vi "задача 3.1.vi"() -> ()   [LabVIEW 2019]
uses:
  <vilib>/Utility/file.llb/Read Delimited Spreadsheet (I64).vi
panel:
  out "Min":dbl
  out "Max":dbl
  in  "Path":path
  out "Waveform Chart":i64[](graph)
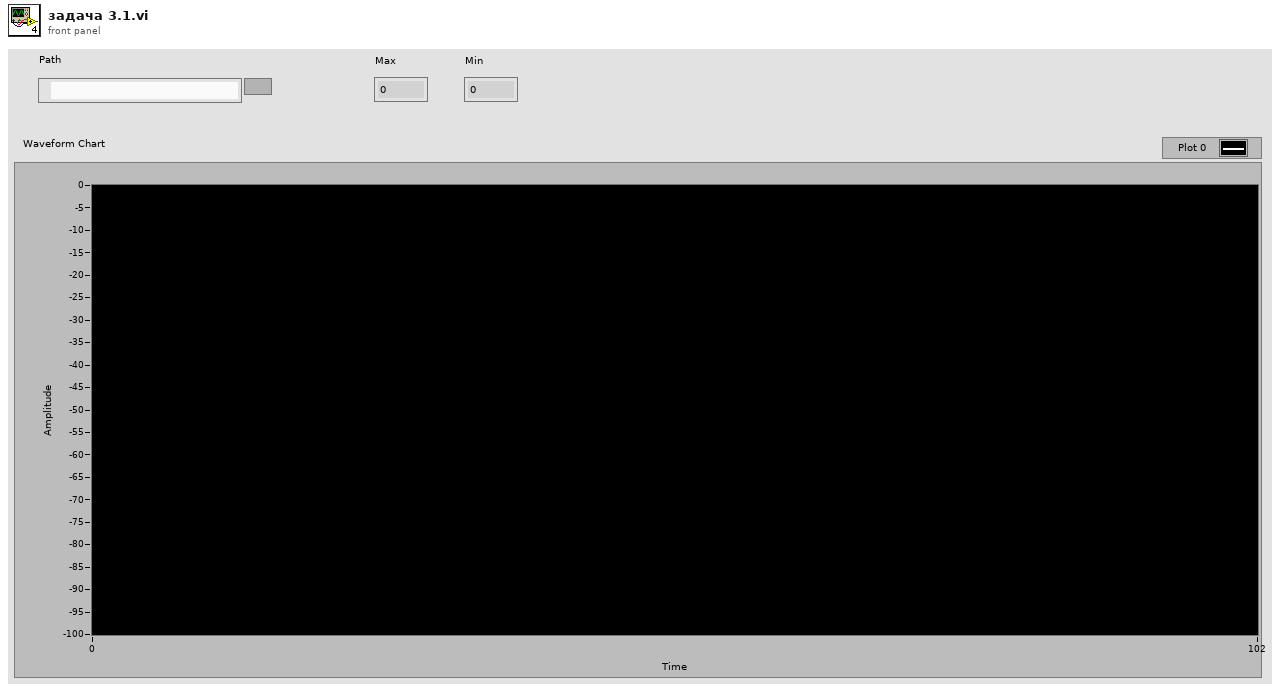
[diagram p1: front panel]
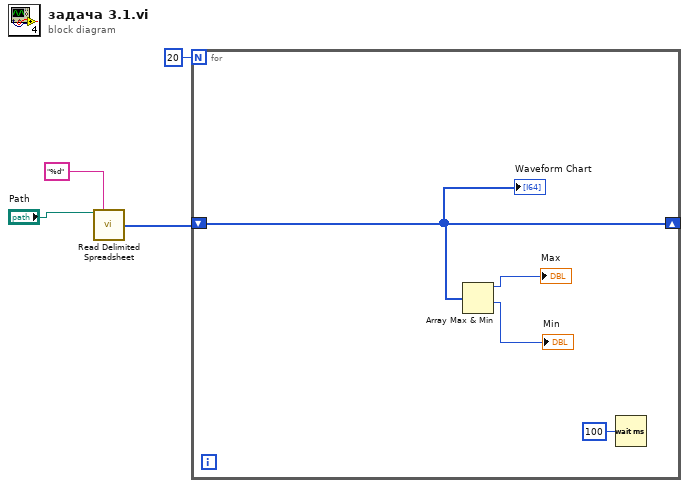
[diagram p0: block diagram]
diagram:
  n1 = call-poly <vilib>:"Read Delimited Spreadsheet.vi"("file path (dialog if empty)"="Path", "format (%d)"="%d") -> ("first row"=w1:i64[])  [unwired: 8 in, 5 out]
  n2 = for {
    N: 20 -> [_]
    shift-right: [w7] -> _
    shift-left: w1 -> [w7]
    n3 = Array Max & Min(array=w7) -> (max value=→"Max":i64, min value=→"Min":i64)  [unwired: 2 out]
    n4 = Wait (ms)(milliseconds to wait=u32 100) -> ()  [unwired: 1 out]
    "Waveform Chart" <- w7
  }
